vi "Reset Time Counter.vi"(8 "Error In (no error)":errorcluster, 11 "VISA Resource Name":refnum<visa-resource-name>) -> (0 "Error Out":errorcluster, 3 "VISA Resource Name Out":refnum<visa-resource-name>)   [LabVIEW 2010, in "Stanford Research 844.lvlib"]
doc: "This VI resets the time counter."
uses:
  <instrlib>/Stanford Research 844/Stanford Research 844.lvlib
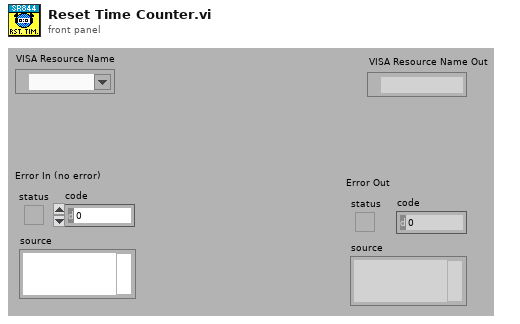
[diagram p1: front panel]
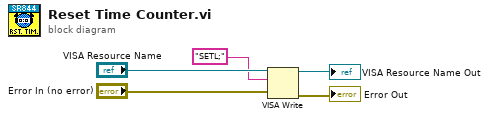
[diagram p0: block diagram]
diagram:
  n1 = VISA Write(VISA resource name="VISA Resource Name", write buffer="SETL;" ("true string"), error in (no error)="Error In (no error)") -> (VISA resource name out=→"VISA Resource Name Out":refnum<visa-resource-name>, error out=→"Error Out":errorcluster)  [unwired: 1 out]
